vi "Get Master RIO.vi"(8 "error in (no error)":errorcluster, 11 "EST Custom Device in":refnum<k24>) -> (0 "error out":errorcluster, 2 "RIO Device Address":string, 3 "EST Custom Device out":refnum<k24>)   [LabVIEW 2015, in "Engine Simulation Toolkit Scripting API.lvlib"]
uses:
  Engine Simulation Toolkit Scripting API.lvlib
  NationalInstruments.VeriStand.SystemDefinitionAPI
  Shared/Properties.vi
  <vilib>/NI Veristand/Custom Device API/Get Item Property (String).vi
  Shared/Engine Simulation Toolkit Shared.lvlib
  <vilib>/NI VeriStand/Custom Device API/Custom Device API.lvlib
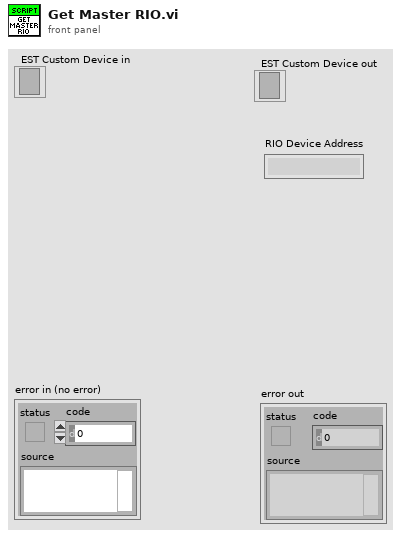
[diagram p1: front panel]
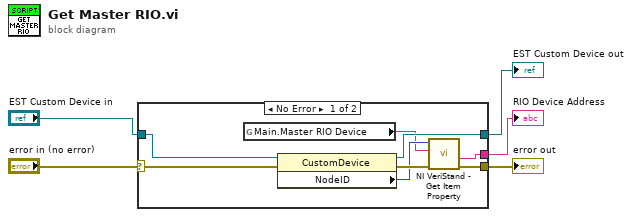
[diagram p0: block diagram]
diagram:
  n1 = case shown="No Error" "error in (no error)" {
    selector: "error in (no error)" -> [w12 w15]
    tunnel: [w10 w15] -> w5
    tunnel: "EST Custom Device in" -> [w13 w14]
    tunnel: [w11 w14] -> w2
    tunnel: [w6 _] -> w1
    frame No Error {
      n2 = global read "Properties.vi" "Main.Master RIO Device"() -> (w7:string)
      n3 = property class="CustomDevice"(reference=w13, error in=w12) -> (reference out=w11:refnum<k24>, error out=w9:errorcluster, "NodeID"=w8:u64)
      n4 = call-poly <vilib>:"NI VeriStand - Get Item Property.vi"("error in (no error)"=w9, "Property Name"=w7, "Item Ref in"=w8) -> ("error out"=w10:errorcluster, "Value"=w6:string)  [unwired: 5 in, 2 out]
    }
    frame Error {
    }
  }
  "EST Custom Device out" <- w2
  "error out" <- w5
  "RIO Device Address" <- w1
